vi "NTV_Max Traverse Speed.vi"(7 "Read(f) Write(t)":bool, 11 "MAx Tavers Speed FPS":dbl=10.0) -> (3 "MAx Traverse Speed FPS Out":dbl)   [LabVIEW 2023]
uses:
  <vilib>/Rock Robotics/Network Tables/NT Read Number.vi
  <vilib>/Rock Robotics/Network Tables/NT Write Number.vi
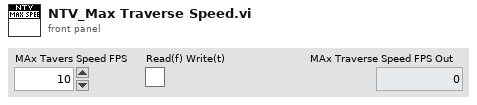
[diagram p1: front panel]
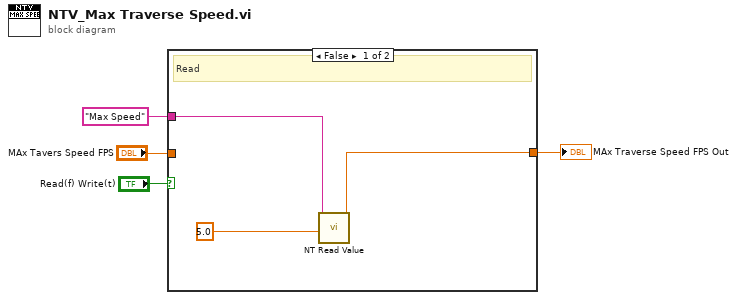
[diagram p0: block diagram]
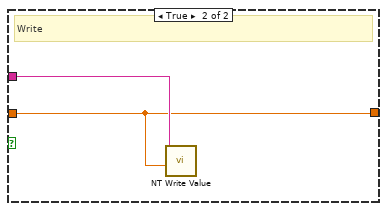
[diagram p2: hidden frame]
diagram:
  n1 = case shown="False" "Read(f) Write(t)" {
    tunnel: "MAx Tavers Speed FPS" -> [_ w8]
    tunnel: "Max Speed" ("Name") -> [w7 w9]
    tunnel: [w5 w8] -> w1
    frame False {
      # "Read"
      n2 = call-poly <vilib>:"NT Read Value.vi"("default value"=5.0 ("Default Value"), "name"=w7) -> ("value"=w5:dbl)  [unwired: 7 in, 2 out]
    }
    frame True {
      # "Write"
      n3 = call-poly <vilib>:"NT Write Value.vi"("value"=w8, "name"=w9) -> ()  [unwired: 9 in, 1 out]
    }
  }
  "MAx Traverse Speed FPS Out" <- w1
